vi "regStopServerOcc.vi"(8 "error in (no error)":errorcluster, 11 "tcpServerBase in":refnum<class "TcpServerBase.lvclass">) -> (0 "error out":errorcluster, 3 "tcpServerBase out":refnum<class "TcpServerBase.lvclass">)   [LabVIEW 2018, in "TcpServerBase.lvclass"]
doc: "Register the stopServer occurrence. This occurrence will be used to stop all servers."
uses:
  TcpServerBase.lvclass
  TcpServerBase.lvclass/TcpServerBase.ctl
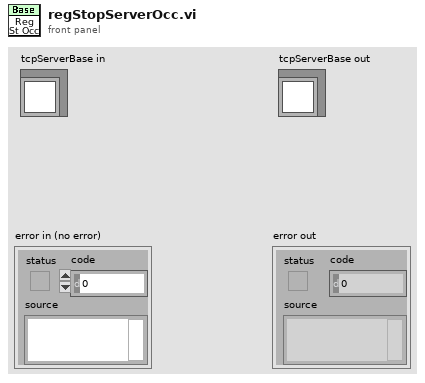
[diagram p1: front panel]
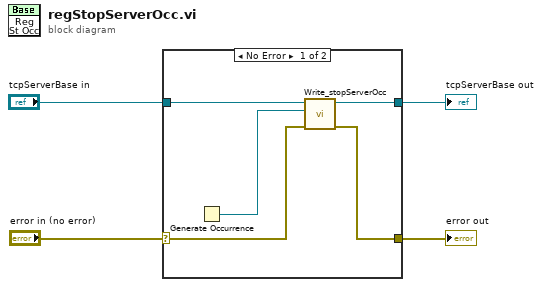
[diagram p0: block diagram]
diagram:
  n1 = case shown="No Error" "error in (no error)" {
    selector: "error in (no error)" -> [w6 w11]
    tunnel: [w7 w11] -> w3
    tunnel: [w8 w10] -> w1
    tunnel: "tcpServerBase in" -> [w9 w10]
    frame No Error {
      n2 = Generate Occurrence() -> (w5:refnum<k4>)
      n3 = call "Write_stopServerOcc.vi"("error in (no error)"=w6, "stopServerOcc"=w5, "TcpServerBase in"=w9) -> ("error out"=w7:errorcluster, "TcpServerBase out"=w8:refnum<class "TcpServerBase.lvclass">)  [unwired: 7 in]
    }
    frame Error {
    }
  }
  "error out" <- w3
  "tcpServerBase out" <- w1
